vi "voltage_out_test.vi"() -> ()   [LabVIEW 2014]
uses:
  <vilib>/DAQmx/write.llb/DAQmx Write (Analog 1D DBL 1Chan NSamp).vi
  <vilib>/DAQmx/create/channels.llb/DAQmx Create Channel (AO-Voltage-Basic).vi
  <vilib>/DAQmx/configure/timing.llb/DAQmx Timing (Sample Clock).vi
  <vilib>/DAQmx/miscellaneous.llb/DAQmx Fill In Error Info.vi
  <resource>/objmgr/daqmx.rc
panel:
  in  "Knob Control or Sine Wave 0ß10V":bool
  in  "stop (F)":bool caption="stop Sine Wave"
  out "error message":string=" INSTRUCTIONS:\r\rNormal Use:  When using subVIs that incorporate the error in/error out (or error I/O) structure, place this handler where you want to inform the user of an error, typically at the end of the I/O data path, as the last action of the program.  If the error in error? is ERROR, the handler creates a message describing the error and its source.  If the type of dialog = 1 (default), the message is displayed to the user, who can only acknowedge it.  If the type = 2, the user can acknowledge the message or abort execution; aborting a program with active I/O is not recommended.  If the type = 0, no message is displayed; this is used to process the error programmatically, and the error out cluster elements are wired to individual terminals for that reason.  \r\rOther Use:\n\r\nlocal testing.  To test the error code of a subVI or function that does not have the error I/O structure, you can wire its error code and a source string to the local error code and error source inputs.  If error in error? indicates no error and error code is not equal to 0, the local code and source are substituted for the error in values, and error? is set TRUE (ERROR)."
  in  "DAQmx Physical Channel":tag="Dev1/ao0"
  in  "state":string="Acquiring Data..."
  in  "current P_rad sample":dbl(knob) scale=0.0..10.0
  in  "Stop Voltage Output":bool
  in  "sample mode":i32(ring)=10123 items=["Finite Samples"=10178, "Continuous Samples"=10123, "Hardware Timed Single Point"=12522]
  in  "RegenMode":i32(ring)=10158 items=["Allow Regeneration"=10097, "Do Not Allow Regeneration"=10158]
  in  "rate of voltage sampling":dbl=100000.0 format="%#_13g"
  out "number of samples written on channel":u32
  out "number of samples per iteration":dbl
  in  "maximum voltage @ 10MW":dbl=5.0 format="%#_13g"
  # "Sine Wave Controls"
  # "Knob Controls"
  # "Acquiring Data... = Running\n\nAcquiring done = Stop"
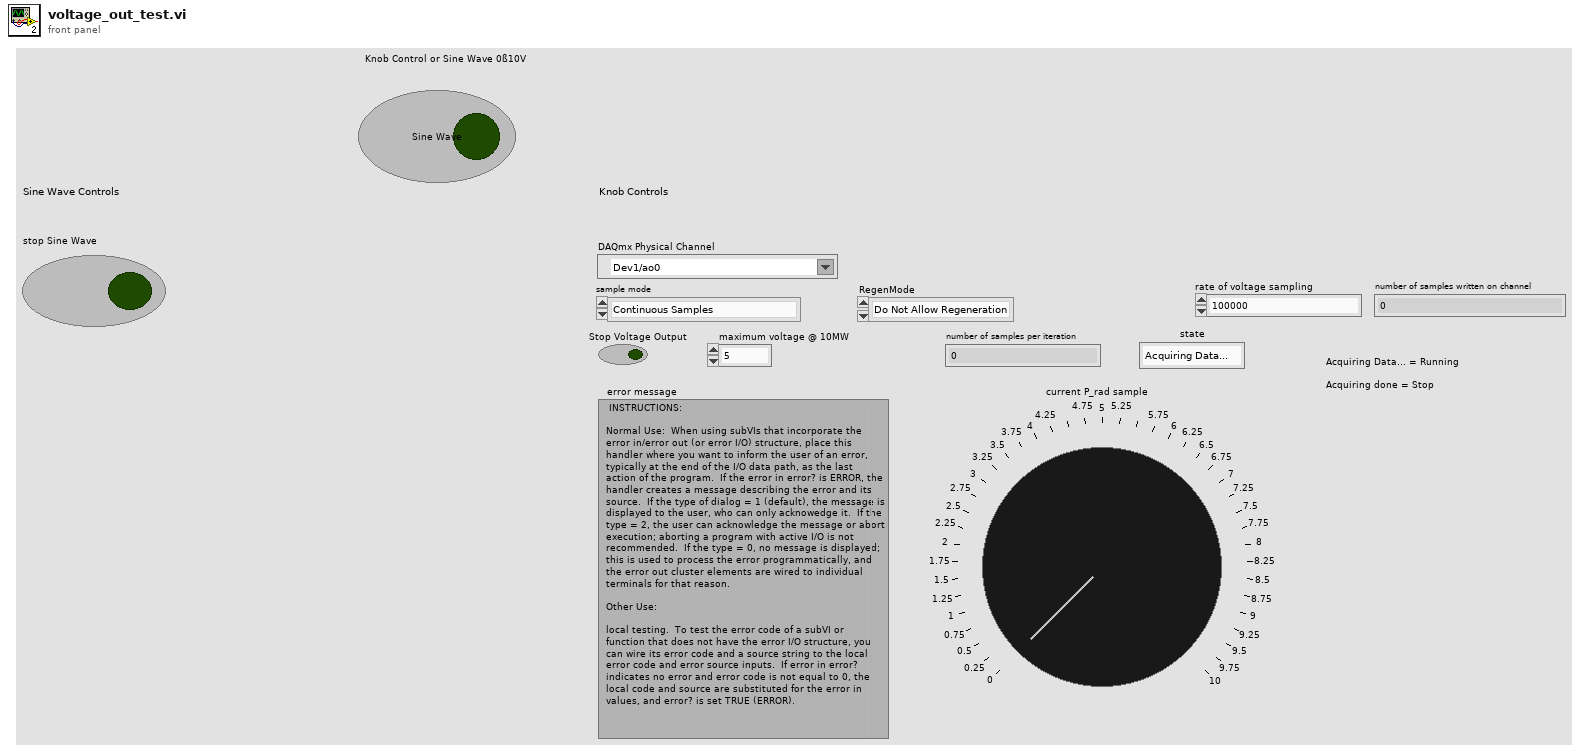
[diagram p1: front panel]
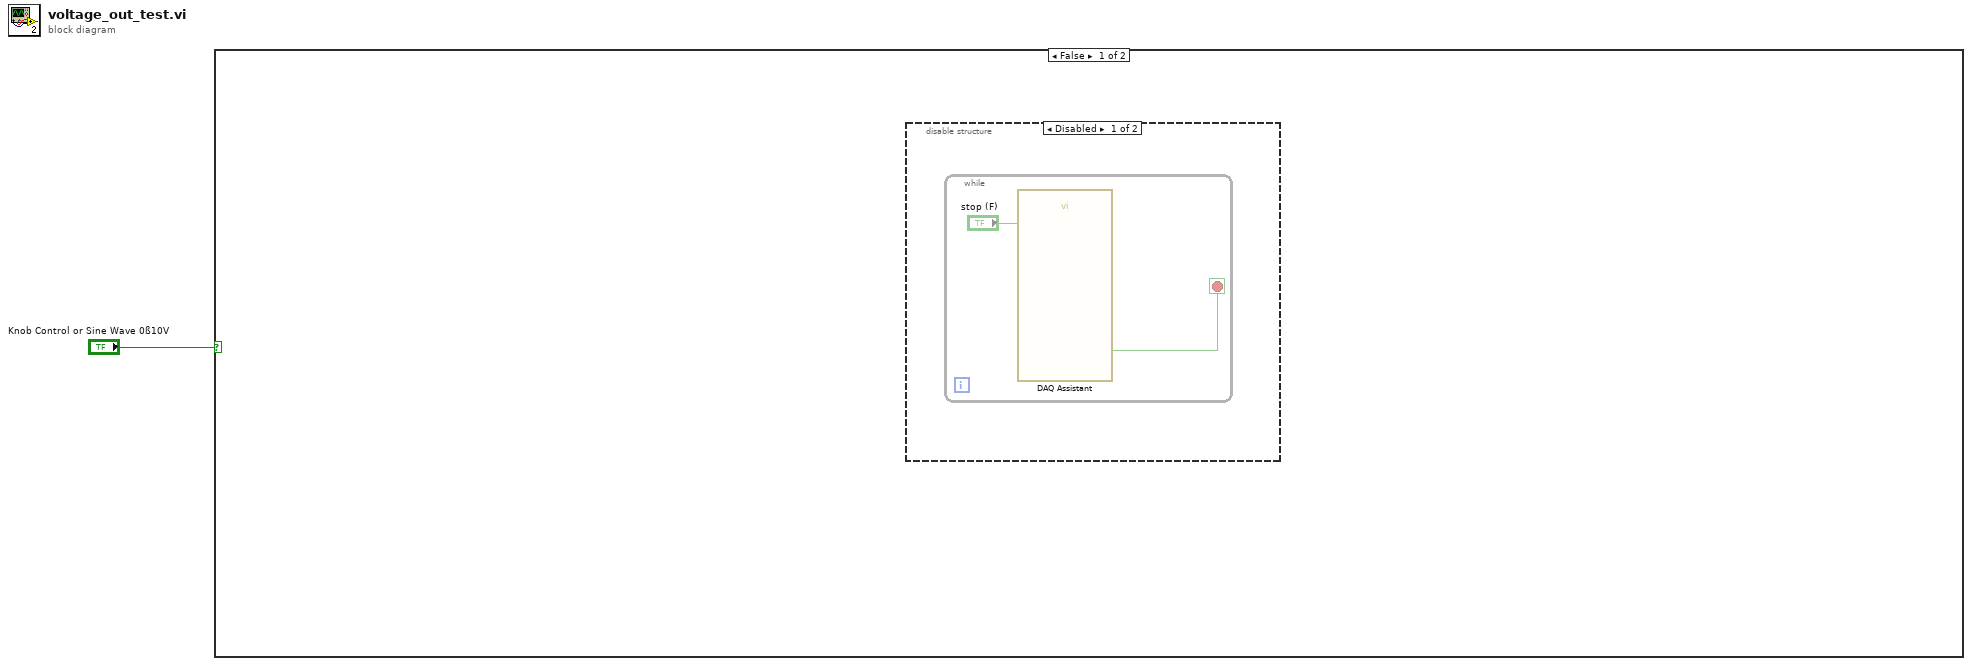
[diagram p0: block diagram]
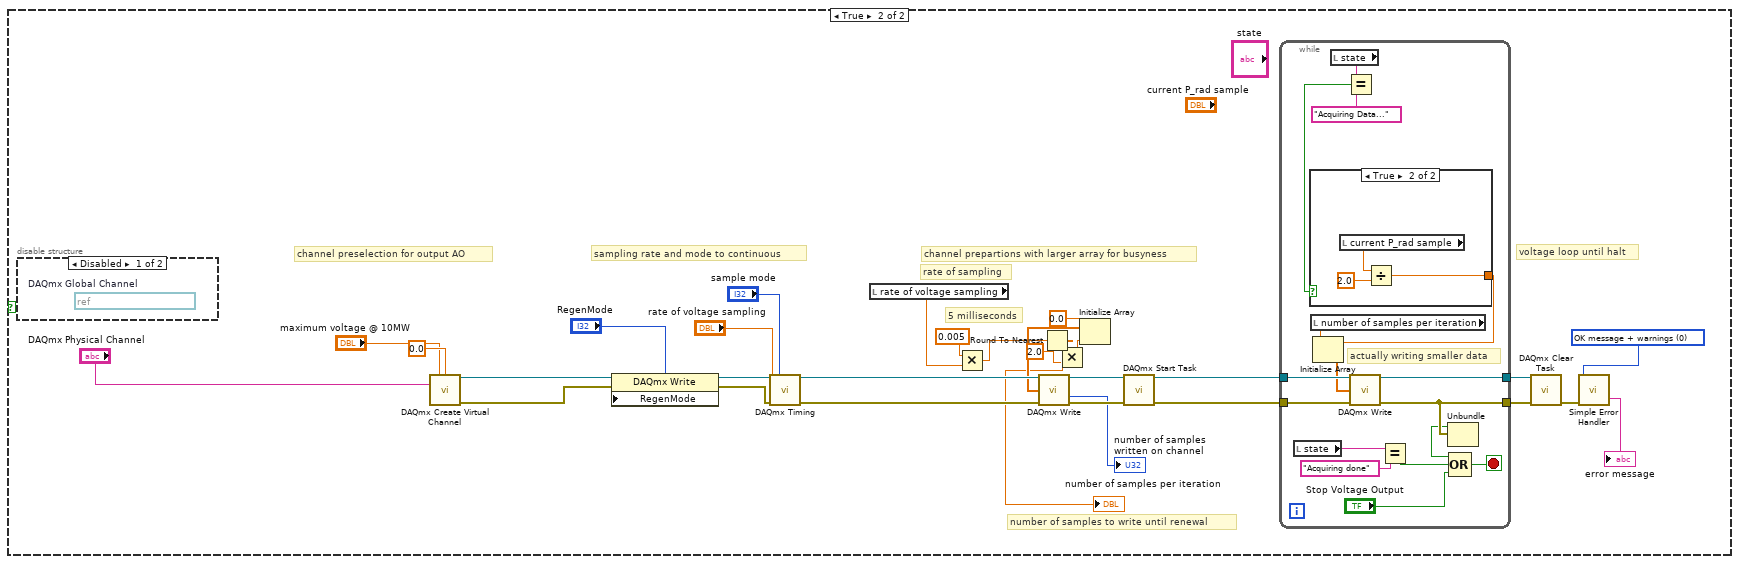
[diagram p3: hidden frame]
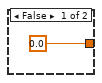
[diagram p5: hidden frame]
diagram:
  n1 = case shown="False" "Knob Control or Sine Wave 0ß10V" {
    frame False {
      n2 = disable-structure shown="Disabled" {
        frame Disabled {
          n3 = while {
            stop <- w2 stop-if-true
            n4 = call "DAQ Assistant"("stop (F)"="stop (F)") -> ("stopped"=w2:bool)  [unwired: 16 in, 2 out]
          }
        }
        frame Enabled {
        }
      }
    }
    frame True {
      w29 = u16 0 items=["OK message + warnings"]
      # "voltage loop until halt"
      # "channel prepartions with larger array for busyness"
      # "sampling rate and mode to continuous"
      # "channel preselection for output AO"
      # "number of samples to write until renewal"
      # "rate of sampling"
      # "5 milliseconds"
      n5 = disable-structure shown="Disabled" {
        frame Disabled {
          (unwired) refnum<k21> "VoltageOutChannel"  # DAQmx Global Channel
        }
        frame Enabled {
        }
      }
      n6 = call-poly <vilib>:"DAQmx Create Virtual Channel.vi"("maximum value"="maximum voltage @ 10MW", "minimum value"=0.0, "physical channels"="DAQmx Physical Channel") -> ("task out"=w26:refnum<k21>, "error out"=w25:errorcluster)  [unwired: 11 in]
      n7 = property class="DAQmx Write"(reference=w26, error in=w25, "RegenMode"="RegenMode") -> (reference out=w24:refnum<k21>, error out=w22:errorcluster)
      n8 = call-poly <vilib>:"DAQmx Timing.vi"("task/channels in"=w24, "sample mode"="sample mode", "rate"="rate of voltage sampling", "error in"=w22) -> ("task out"=w21:refnum<k21>, "error out"=w19:errorcluster)  [unwired: 10 in]
      n9 = local read "rate of voltage sampling"() -> (w16:dbl)
      n10 = Multiply(x=0.005, y=w16) -> (x*y=w10:dbl)
      n11 = Round To Nearest(number=w10) -> (nearest integer value=w8:dbl)
      "number of samples per iteration" <- w8
      n12 = Multiply(x=w8, y=2.0) -> (x*y=w7:dbl)
      n13 = Initialize Array(0.0 ("element"), w7) -> (w18:dbl[])
      n14 = call-poly <vilib>:"DAQmx Write.vi"("task/channels in"=w21, "data"=w18, "error in"=w19) -> ("task out"=w15:refnum<k21>, "number of samples written per channel"=→"number of samples written on channel":u32, "error out"=w14:errorcluster)  [unwired: 10 in]
      n15 = call <vilib>:"DAQmx Start Task.vi"("task/channels in"=w15, "error in"=w14) -> ("task out"=w12:refnum<k21>, "error out"=w11:errorcluster)  [unwired: 12 in]
      n16 = while {
        tunnel: w11 -> [w48]
        tunnel: [w38] -> w31
        tunnel: w12 -> [w49]
        tunnel: [w47] -> w32
        stop <- w34 stop-if-true
        # "actually writing smaller data"
        n17 = local read "state"() -> (w40:string)
        n18 = local read "number of samples per iteration"() -> (w43:dbl)
        n19 = local read "state"() -> (w46:string)
        n20 = Equal?(x=w46, y="Acquiring Data...") -> (x = y?=w44:bool)
        n21 = case shown="True" w44 {
          tunnel: [0.0 w51] -> w42
          frame False {
          }
          frame True {
            n22 = local read "current P_rad sample"() -> (w52:dbl)
            n23 = Divide(x=w52, y=2.0) -> (x/y=w51:dbl)
          }
        }
        n24 = Initialize Array(w42, w43) -> (w41:dbl[])
        n25 = call-poly <vilib>:"DAQmx Write.vi"("task/channels in"=w49, "data"=w41, "error in"=w48) -> ("task out"=w47:refnum<k21>, "error out"=w38:errorcluster)  [unwired: 10 in, 1 out]
        n26 = Equal?(x=w40, y="Acquiring done" ("state")) -> (x = y?=w36:bool)
        n27 = Unbundle(w38) -> ("status"=w37:bool)  [unwired: 2 out]
        n28 = Compound Arithmetic op=OR(w37, w36, "Stop Voltage Output") -> (w34:bool)
      }
      n29 = call <vilib>:"DAQmx Clear Task.vi"("task in"=w32, "error in"=w31) -> ("error out"=w30:errorcluster)  [unwired: 13 in]
      n30 = call <vilib>:"Simple Error Handler.vi"("type of dialog (OK msg:1)"=w29, "error in (no error)"=w30) -> ("message"=→"error message":string)  [unwired: 3 in, 4 out]
    }
  }
